vi "Alarm Cluster to Alarm Model Cluster.vi"(10 "Alarm Name":string="TT1:Lo", 11 "Alarm":T2={"alarm URL"="\\\\Nate-VM-LV2018\\Pfizer FAST\\TT1.Alarms.TT1:Lo", "set time"=timestamp(3634824639.8324924 s since 1904-01-01), "set user"="(Nobody)", "ack time"=timestamp(-9223372036854775808 s since 1904-01-01), "ack user"="", "clear time"=timestamp(-9223372036854775808 s since 1904-01-01), "clear user"="", "setpoint"=30.0, "value"=22.498404260798484, "priority"=1, "alarm area"="", "alarm description"="", "ack comment"="", "event?"=FALSE, "Refnum"=216172782113783883} {"value" format="%.2f"; "setpoint" format="%.2f"; "clear time" format="%<%X\n%x>T"; "ack time" format="%<%X\n%x>T"; "set time" format="%<%X\n%x>T"}) -> (3 "Alarm Model":T1={"Color Box"=16777226, "Name"="TT1:Lo", "Ack"=FALSE, "Alarm"={"alarm URL"="\\\\.\\Pfizer FAST\\TT1.Alarms.TT1:Lo", "set time"=timestamp(3634824639.8324924 s since 1904-01-01), "set user"="(Nobody)", "ack time"=timestamp(-9223372036854775808 s since 1904-01-01), "ack user"="", "clear time"=timestamp(-9223372036854775808 s since 1904-01-01), "clear user"="", "setpoint"=30.0, "value"=22.498404260798484, "priority"=1, "alarm area"="", "alarm description"="", "ack comment"="", "event?"=FALSE, "Refnum"=216172782113783883}} {"Alarm"."value" format="%.2f"; "Alarm"."setpoint" format="%.2f"; "Alarm"."clear time" format="%<%X\n%x>T"; "Alarm"."ack time" format="%<%X\n%x>T"; "Alarm"."set time" format="%<%X\n%x>T"})   [LabVIEW 2018, in "Dynamic Shared Variables.lvlib"]
doc: "Given Alarm information, save the data that we need to display a nice alarm indicator into the \"Alarm Model\"."
uses:
  Dynamic Shared Variables.lvlib
  Alarm Cluster.ctl
panel:
  out "acknowledged?":bool=TRUE
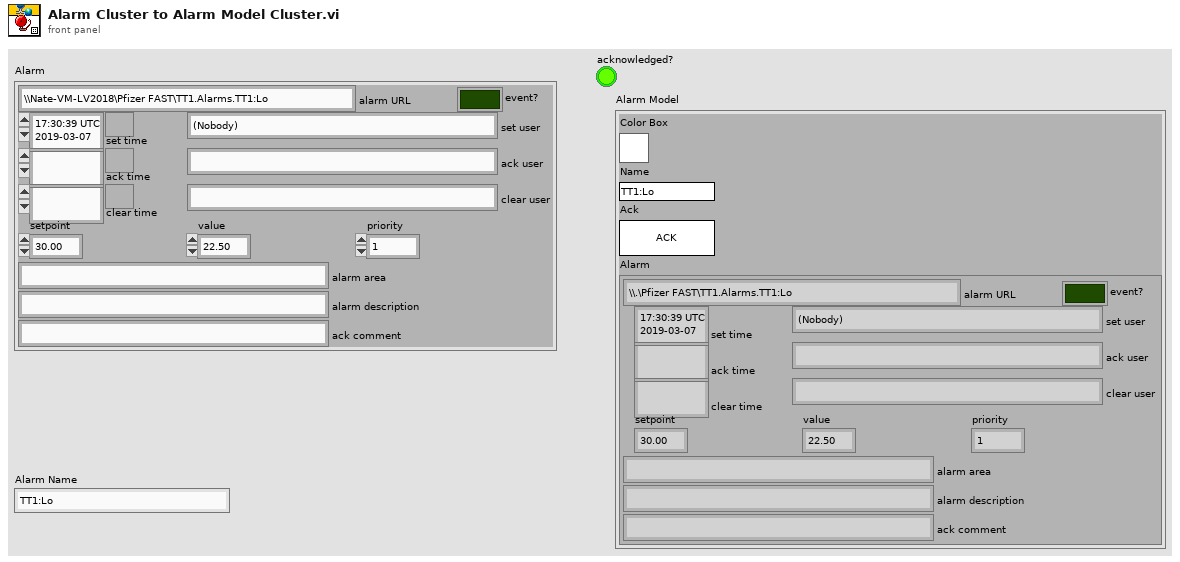
[diagram p1: front panel]
types:
  T1 = typedef "Dynamic Shared Variables.lvlib/Alarm Cluster.ctl" = cluster{"Color Box":u32, "Name":string, "Ack":bool, "Alarm":cluster{"alarm URL":string, "set time":timestamp, "set user":string, "ack time":timestamp, "ack user":string, "clear time":timestamp, "clear user":string, "setpoint":dbl, "value":dbl, "priority":u32, "alarm area":string, "alarm description":string, "ack comment":string, "event?":bool, "Refnum":u64}}
  T2 = cluster{"alarm URL":string, "set time":timestamp, "set user":string, "ack time":timestamp, "ack user":string, "clear time":timestamp, "clear user":string, "setpoint":dbl, "value":dbl, "priority":u32, "alarm area":string, "alarm description":string, "ack comment":string, "event?":bool, "Refnum":u64}
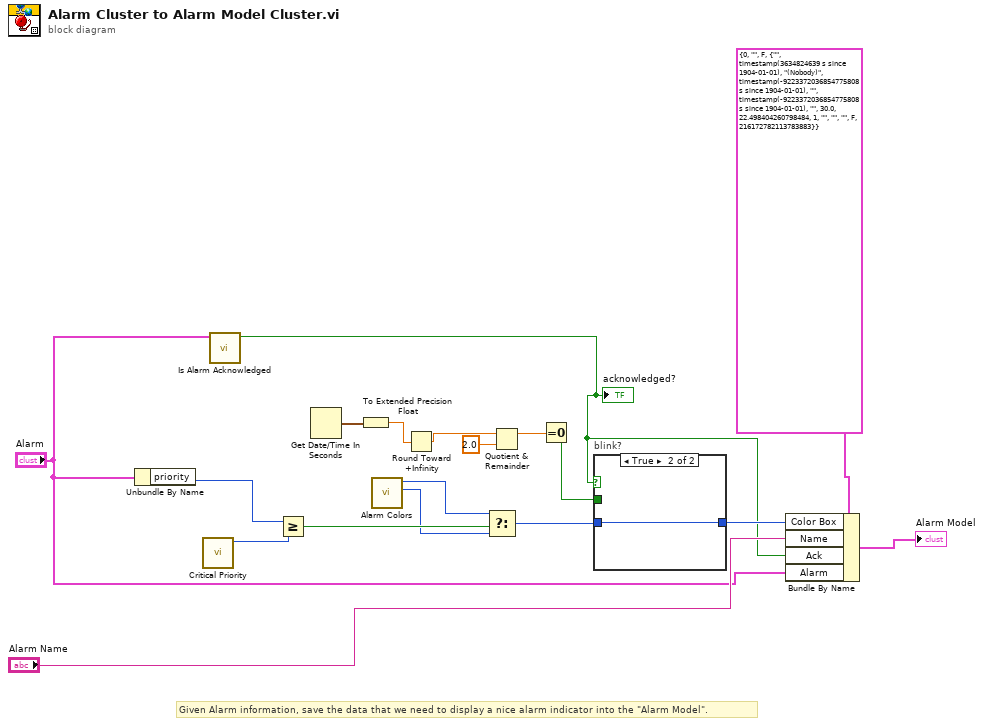
[diagram p0: block diagram]
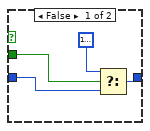
[diagram p2: hidden frame]
diagram:
  # "Given Alarm information, save the data that we need to display a nice alarm indicator into the \"Alarm Model\"."
  n1 = Unbundle By Name("Alarm") -> ("priority"=w15:u32)
  n2 = call "Critical Priority.vi"() -> ("critical priority"=w18:i32)  [unwired: 11 in]
  n3 = call "Is Alarm Acknowledged.vi"("Alarm"="Alarm") -> ("Acknowledged?"=w1:bool)  [unwired: 8 in, 2 out]
  "acknowledged?" <- w1
  n4 = Greater Or Equal?(x=w15, y=w18) -> (x >= y?=w14:bool)
  n5 = Get Date/Time In Seconds() -> (seconds since 1Jan1904=w6:timestamp)
  n6 = To Extended Precision Float(1:w6) -> (0:w5:ext)
  n7 = call "Alarm Colors.vi"() -> ("Non-critical"=w2:u32, "Critical"=w3:u32)  [unwired: 10 in]
  n8 = Round Toward +Infinity(x=w5) -> (ceil(x): smallest int >= x=w13:ext)
  n9 = Select(t=w3, s=w14, f=w2) -> (s? t:f=w9:u32)
  n10 = Quotient & Remainder(x=w13, y=2.0) -> (x-y*floor(x/y)=w11:ext)  [unwired: 1 out]
  n11 = Equal To 0?(x=w11) -> (x = 0?=w8:bool)
  n12 = case "blink?" shown="True" w1 {
    tunnel: [w19 w23] -> w10
    tunnel: w9 -> [w21 w23]
    tunnel: w8 -> [w22 _]
    frame False {
      n13 = Select(t=u32 16777226, s=w22, f=w21) -> (s? t:f=w19:u32)
    }
    frame True {
    }
  }
  n14 = Bundle By Name(cluster=T1 {"Color Box"=0, "Name"="", "Ack"=FALSE, "Alarm"={"alarm URL"="", "set time"=timestamp(3634824639.8324924 s since 1904-01-01), "set user"="(Nobody)", "ack time"=timestamp(-9223372036854775808 s since 1904-01-01), "ack user"="", "clear time"=timestamp(-9223372036854775808 s since 1904-01-01), "clear user"="", "setpoint"=30.0, "value"=22.498404260798484, "priority"=1, "alarm area"="", "alarm description"="", "ack comment"="", "event?"=FALSE, "Refnum"=216172782113783883}} ("Alarm Cluster"), "Color Box"=w10, "Name"="Alarm Name", "Ack"=w1, "Alarm"="Alarm") -> (→"Alarm Model":T1)
